vi "TDMS Advanced - Write Asynchronously.vi"   [LabVIEW 2020]
panel:
  # "For instructions, select Help>>Show Context Help and move the cursor over the VI icon to display help for this VI."
types:
  T1 = enum16{"open", "open or create", "create or replace", "create", "open (read-only)"}
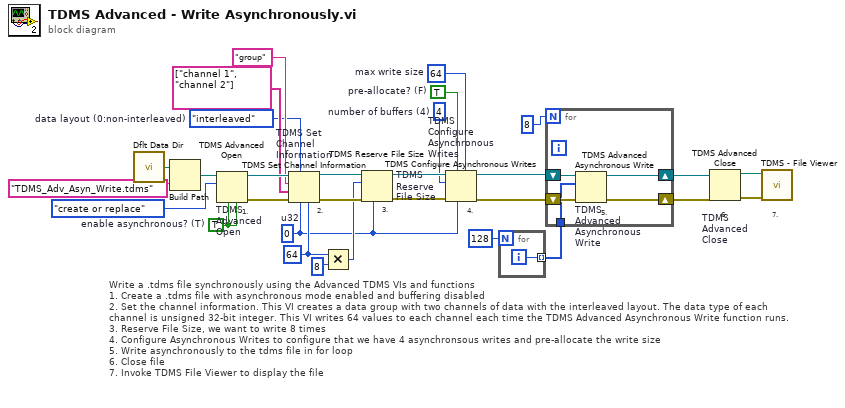
[diagram p0: block diagram]
diagram:
  w1 = u32 64  # max write size
  w2 = TRUE  # pre-allocate? (F)
  w5 = u32 4  # number of buffers (4)
  w12 = TRUE  # enable asynchronous? (T)
  w4 = u32 64 ("samples per channel")
  w3 = u32 0  # u32
  w22 = enum16{"non-interleaved", "interleaved"}."interleaved"  # data layout (0:non-interleaved)
  # "4."
  # "Write a .tdms file synchronously using the Advanced TDMS VIs and functions\n1. Create a .tdms file with asynchronous mode enabled and buffering disabled\n2. Set the channel information. This VI creates a data group with two channels of data with the interleaved layout. The data type of each channel is unsigned 32-bit integer. This VI writes 64 values to each channel each time the TDMS Advanced Asynchronous Write function runs.\n3. Reserve File Size, we want to write 8 times\n4. Configure Asynchronous Writes to configure that we have 4 asynchronsous writes and pre-allocate the write size \n5. Write asynchronously to the tdms file in for loop\n6. Close file\n7. Invoke TDMS File Viewer to display the file"
  # "7."
  # "1."
  # "6."
  # "3."
  # "2."
  n1 = call <vilib>:"Dflt Data Dir.vi"() -> ("App:Default Data Directory"=w25:path)
  n2 = Build Path(base path=w25, name or relative path="TDMS_Adv_Asyn_Write.tdms") -> (appended path=w29:path)
  n3 = TDMS Advanced Open "TDMS\nAdvanced\nOpen"(4:w12, 6:w12, 10:T1."create or replace" ("operation (0:open)"), 11:w29) -> (0:w27:errorcluster, 3:w26:refnum<k34>)  [unwired: 1 in, 1 out]
  n4 = TDMS Set Channel Information "TDMS Set\nChannel\nInformation"(4:w4, 6:w3, 7:w22, 8:w27, 9:string[] ["channel 1", "channel 2"] ("channel name(s)"), 10:"group" ("group name (Untitled)"), 11:w26) -> (0:w16:errorcluster, 3:w15:refnum<k34>)
  n5 = Multiply(x=w4, y=u32 8) -> (x*y=w13:u32)
  n6 = TDMS Reserve File Size "TDMS\nReserve\nFile Size"(6:w3, 8:w16, 10:w13, 11:w15) -> (0:w9:errorcluster, 3:w8:refnum<k34>)  [unwired: 1 in]
  n7 = TDMS Configure Asynchronous Writes "TDMS\nConfigure\nAsynchronous\nWrites"(5:w1, 6:w3, 7:w2, 8:w9, 10:w5, 11:w8) -> (0:w6:errorcluster, 3:w7:refnum<k34>)  [unwired: 1 in]
  n8 = for {
    N: 128 -> [_]
    tunnel: [w31] -> w19 mode=indexing
    i -> [w31]
  }
  n9 = for {
    N: 8 -> [_]
    shift-right: [w33] -> w17
    shift-left: w7 -> [w35]
    shift-right: [w34] -> w18
    shift-left: w6 -> [w36]
    tunnel: w19 -> [w32]
    # "5."
    n10 = TDMS Advanced Asynchronous Write "TDMS\nAdvanced\nAsynchronous\nWrite"(8:w36, 10:w32, 11:w35) -> (0:w34:errorcluster, 3:w33:refnum<k34>)
  }
  n11 = TDMS Advanced Close "TDMS\nAdvanced\nClose"(8:w18, 11:w17) -> (0:w11:errorcluster, 3:w10:path)  [unwired: 2 in]
  n12 = call <vilib>:"TDMS - File Viewer.vi"("error in (no error)"=w11, "file path"=w10) -> ()  [unwired: 4 in, 2 out]
